vi "Event-MouseWheel.vi"(8 "error in (no error)":errorcluster, 9 "MouseWheelEvent":T1, 10 "EventType":T5=enum."SDL_EVENT_WINDOW_DESTROYED", 11 "DVR Cluster In":T6={"CMD Queue"=refnum, "Config"={"Quit On Last Window Closed"=FALSE, "VSync"=enum."Disabled", "FPS Target"=30.0}, "Ctxt"={"VSync Enabled"=FALSE}, "Metrics"={"Uptime [ms]"=0, "Loop Time [ms]"=0, "Timer [ns]"=0, "Poll Events [ns]"=0, "Dequeue CMD [ns]"=0, "Update Layout [ns]"=0, "Render [ns]"=0}, "Debug"={"Unhandled Events"={}}, "ID To Window"={}, "Window To Handle"={}, "Event Interface"=refnum}) -> (0 "error out":errorcluster, 3 "DVR Cluster Out":T6={"CMD Queue"=refnum, "Config"={"Quit On Last Window Closed"=FALSE, "VSync"=enum."Disabled", "FPS Target"=30.0}, "Ctxt"={"VSync Enabled"=FALSE}, "Metrics"={"Uptime [ms]"=0, "Loop Time [ms]"=0, "Timer [ns]"=0, "Poll Events [ns]"=0, "Dequeue CMD [ns]"=0, "Update Layout [ns]"=0, "Render [ns]"=0}, "Debug"={"Unhandled Events"={}}, "ID To Window"={}, "Window To Handle"={}, "Event Interface"=refnum})   [LabVIEW 2020, in "GLF.lvlib" / "Engine.lvclass"]
uses:
  Engine.lvclass
  EngineEventInterface/EngineEventInterface.lvclass
  Window/Window.lvclass
  Engine.lvclass/Engine.ctl
  <vilib>/Utility/miscctls.llb/LVMapReplaceAction.ctl
  <vilib>/Saukko/LV SDL3/Sources/SDL3/Events/EventType--enum.ctl
  <vilib>/Saukko/LV SDL3/Sources/SDL3/Events/Events.lvlib
  <vilib>/Saukko/LV SDL3/Sources/SDL3/Rect/FPoint--cluster.ctl
  <vilib>/Saukko/LV SDL3/Sources/SDL3/Rect/Rect.lvlib
  VSync--enum.ctl
  Config--cluster.ctl
  Context--cluster.ctl
  Metrics--cluster.ctl
  Command--enum.ctl
  Command--cluster.ctl
  Command--queue.ctl
  <vilib>/Saukko/LV SDL3/Sources/SDL3/Video/WindowID--integer.ctl
  <vilib>/Saukko/LV SDL3/Sources/SDL3/Video/Video.lvlib
  DVR--cluster.ctl
  Debug--cluster.ctl
  <vilib>/Saukko/LV SDL3/Sources/SDL3/Mouse/MouseID--integer.ctl
  <vilib>/Saukko/LV SDL3/Sources/SDL3/Mouse/Mouse.lvlib
  <vilib>/Saukko/LV SDL3/Sources/SDL3/Mouse/MouseWheelDirection--enum.ctl
  <vilib>/Saukko/LV SDL3/Sources/SDL3/Events/MouseWheelEventData--cluster.ctl
  <vilib>/Saukko/LV SDL3/Sources/SDL3/Video/SDL_Window--pointer.ctl
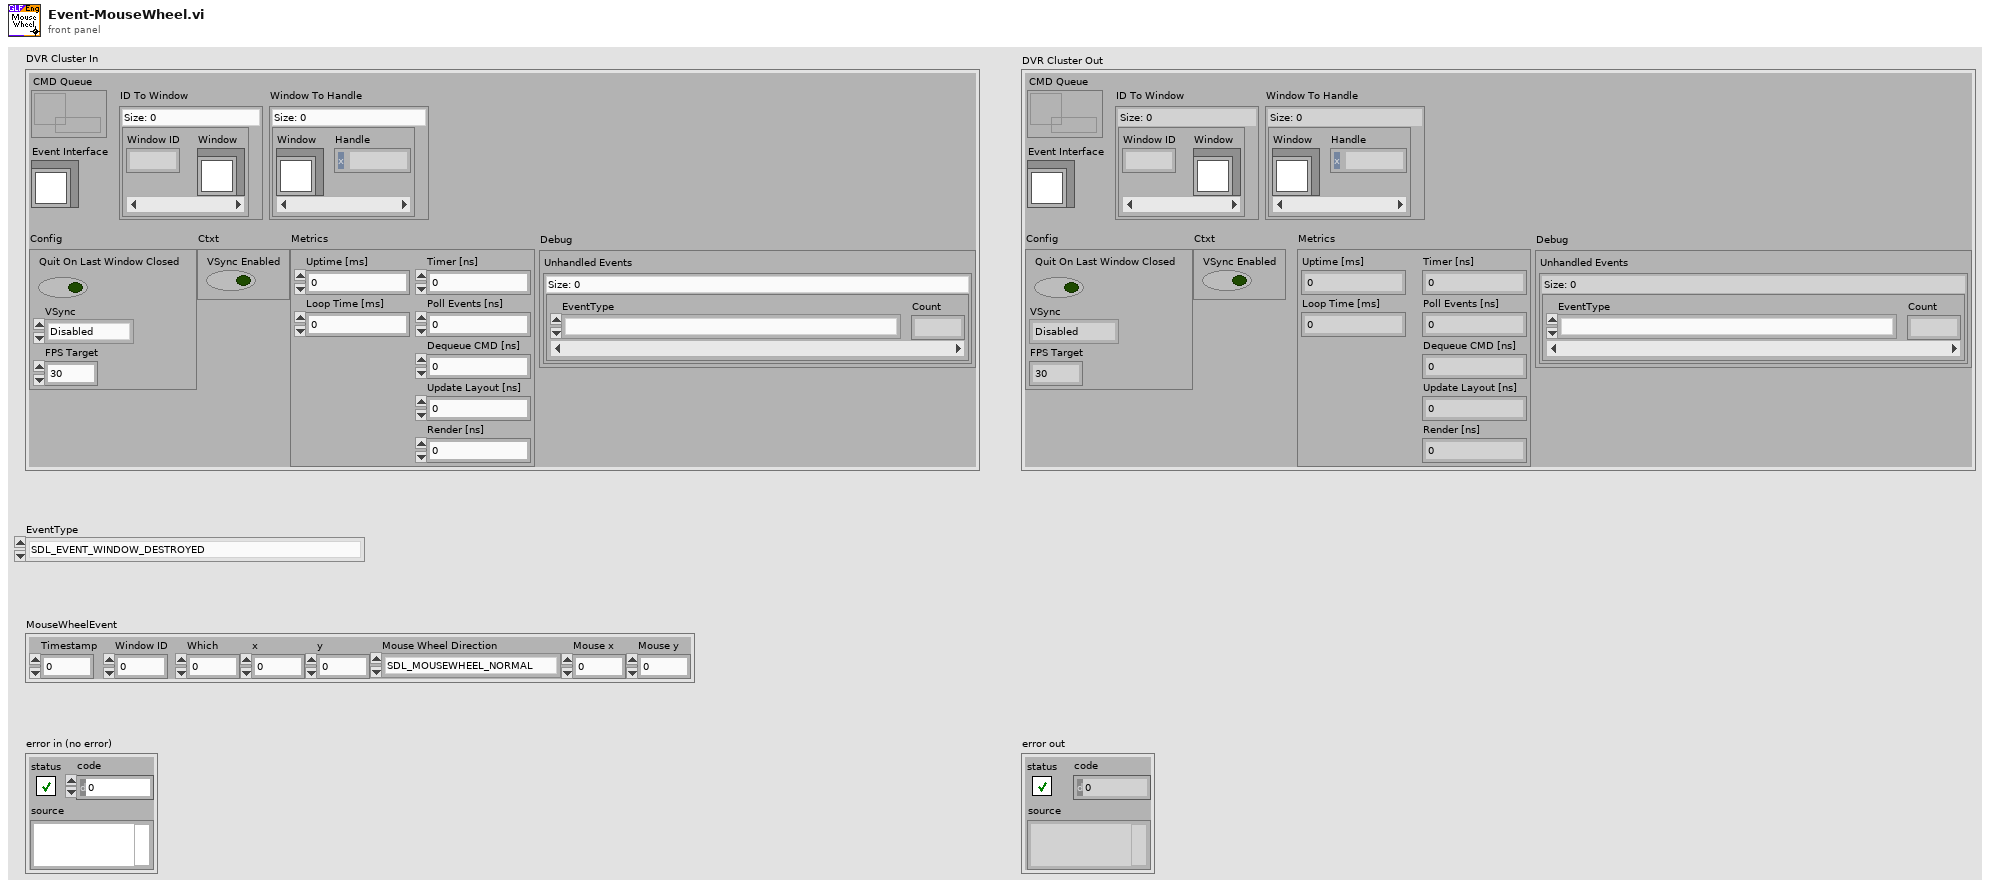
[diagram p1: front panel]
types:
  T1 = typedef "SDL3.lvlib/Events.lvlib/MouseWheelEventData--cluster.ctl" = cluster{"Timestamp":u64, "Window ID":T2, "Which":T3, "x":sgl, "y":sgl, "Mouse Wheel Direction":T4, "Mouse x":sgl, "Mouse y":sgl}
  T2 = typedef "SDL3.lvlib/Video.lvlib/WindowID--integer.ctl" = u32
  T3 = typedef "SDL3.lvlib/Mouse.lvlib/MouseID--integer.ctl" = u32
  T4 = typedef "SDL3.lvlib/Mouse.lvlib/MouseWheelDirection--enum.ctl" = enum32{"SDL_MOUSEWHEEL_NORMAL", "SDL_MOUSEWHEEL_FLIPPED"}
  T5 = typedef "SDL3.lvlib/Events.lvlib/EventType--enum.ctl" = enum16{"LV_NONE", "LV_UNSUPPORTED", "SDL_EVENT_QUIT", "SDL_EVENT_LOCALE_CHANGED", "SDL_EVENT_SYSTEM_THEME_CHANGED", "SDL_EVENT_DISPLAY_ORIENTATION", "SDL_EVENT_DISPLAY_ADDED", "SDL_EVENT_DISPLAY_REMOVED", "SDL_EVENT_DISPLAY_MOVED", "SDL_EVENT_DISPLAY_DESKTOP_MODE_CHANGED", "SDL_EVENT_DISPLAY_CURRENT_MODE_CHANGED", "SDL_EVENT_DISPLAY_CONTENT_SCALE_CHANGED", "SDL_EVENT_WINDOW_SHOWN", "SDL_EVENT_WINDOW_HIDDEN", "SDL_EVENT_WINDOW_EXPOSED", "SDL_EVENT_WINDOW_MOVED", "SDL_EVENT_WINDOW_RESIZED", "SDL_EVENT_WINDOW_PIXEL_SIZE_CHANGED", "SDL_EVENT_WINDOW_METAL_VIEW_RESIZED", "SDL_EVENT_WINDOW_MINIMIZED", "SDL_EVENT_WINDOW_MAXIMIZED", "SDL_EVENT_WINDOW_RESTORED", "SDL_EVENT_WINDOW_MOUSE_ENTER", "SDL_EVENT_WINDOW_MOUSE_LEAVE", "SDL_EVENT_WINDOW_FOCUS_GAINED", "SDL_EVENT_WINDOW_FOCUS_LOST", "SDL_EVENT_WINDOW_CLOSE_REQUESTED", "SDL_EVENT_WINDOW_HIT_TEST", "SDL_EVENT_WINDOW_ICCPROF_CHANGED", "SDL_EVENT_WINDOW_DISPLAY_CHANGED", "SDL_EVENT_WINDOW_DISPLAY_SCALE_CHANGED", "SDL_EVENT_WINDOW_SAFE_AREA_CHANGED", "SDL_EVENT_WINDOW_OCCLUDED", "SDL_EVENT_WINDOW_ENTER_FULLSCREEN", "SDL_EVENT_WINDOW_LEAVE_FULLSCREEN", "SDL_EVENT_WINDOW_DESTROYED", "SDL_EVENT_WINDOW_HDR_STATE_CHANGED", "SDL_EVENT_KEY_DOWN", "SDL_EVENT_KEY_UP", "SDL_EVENT_TEXT_EDITING", "SDL_EVENT_TEXT_INPUT", "SDL_EVENT_KEYMAP_CHANGED", "SDL_EVENT_KEYBOARD_ADDED", "SDL_EVENT_KEYBOARD_REMOVED", "SDL_EVENT_TEXT_EDITING_CANDIDATES", "SDL_EVENT_MOUSE_MOTION", "SDL_EVENT_MOUSE_BUTTON_DOWN", "SDL_EVENT_MOUSE_BUTTON_UP", "SDL_EVENT_MOUSE_WHEEL", "SDL_EVENT_MOUSE_ADDED", "SDL_EVENT_MOUSE_REMOVED", "SDL_EVENT_JOYSTICK_AXIS_MOTION", "SDL_EVENT_JOYSTICK_BALL_MOTION", "SDL_EVENT_JOYSTICK_HAT_MOTION", "SDL_EVENT_JOYSTICK_BUTTON_DOWN", "SDL_EVENT_JOYSTICK_BUTTON_UP", "SDL_EVENT_JOYSTICK_ADDED", "SDL_EVENT_JOYSTICK_REMOVED", "SDL_EVENT_JOYSTICK_BATTERY_UPDATED", "SDL_EVENT_JOYSTICK_UPDATE_COMPLETE", "SDL_EVENT_GAMEPAD_AXIS_MOTION", "SDL_EVENT_GAMEPAD_BUTTON_DOWN", "SDL_EVENT_GAMEPAD_BUTTON_UP", "SDL_EVENT_GAMEPAD_ADDED", "SDL_EVENT_GAMEPAD_REMOVED", "SDL_EVENT_GAMEPAD_REMAPPED", "SDL_EVENT_GAMEPAD_TOUCHPAD_DOWN", "SDL_EVENT_GAMEPAD_TOUCHPAD_MOTION", "SDL_EVENT_GAMEPAD_TOUCHPAD_UP", "SDL_EVENT_GAMEPAD_SENSOR_UPDATE", "SDL_EVENT_GAMEPAD_UPDATE_COMPLETE", "SDL_EVENT_GAMEPAD_STEAM_HANDLE_UPDATED", "SDL_EVENT_FINGER_DOWN", "SDL_EVENT_FINGER_UP", "SDL_EVENT_FINGER_MOTION", "SDL_EVENT_CLIPBOARD_UPDATE", "SDL_EVENT_DROP_FILE", "SDL_EVENT_DROP_TEXT", "SDL_EVENT_DROP_BEGIN", "SDL_EVENT_DROP_COMPLETE", "SDL_EVENT_DROP_POSITION", "SDL_EVENT_AUDIO_DEVICE_ADDED", "SDL_EVENT_AUDIO_DEVICE_REMOVED", "SDL_EVENT_AUDIO_DEVICE_FORMAT_CHANGED", "SDL_EVENT_SENSOR_UPDATE", "SDL_EVENT_PEN_PROXIMITY_IN", "SDL_EVENT_PEN_PROXIMITY_OUT", "SDL_EVENT_PEN_DOWN", "SDL_EVENT_PEN_UP", "SDL_EVENT_PEN_BUTTON_DOWN", "SDL_EVENT_PEN_BUTTON_UP", "SDL_EVENT_PEN_MOTION", "SDL_EVENT_PEN_AXIS", "SDL_EVENT_CAMERA_DEVICE_ADDED", "SDL_EVENT_CAMERA_DEVICE_REMOVED", "SDL_EVENT_CAMERA_DEVICE_APPROVED", "SDL_EVENT_CAMERA_DEVICE_DENIED", "SDL_EVENT_RENDER_TARGETS_RESET", "SDL_EVENT_RENDER_DEVICE_RESET", "SDL_EVENT_POLL_SENTINEL", "SDL_EVENT_USER"}
  T6 = typedef "GLF.lvlib/Engine.lvclass/DVR--cluster.ctl" = cluster{"CMD Queue":T7, "Config":T8, "Ctxt":T10, "Metrics":T11, "Debug":T12, "ID To Window":map{T2, refnum<class "Window.lvclass">}, "Window To Handle":map{refnum<class "Window.lvclass">, T13}, "Event Interface":refnum<class "EngineEventInterface.lvclass">}
  T7 = typedef "GLF.lvlib/Engine.lvclass/Command--queue.ctl" = refnum<queue>
  T8 = typedef "GLF.lvlib/Engine.lvclass/Config--cluster.ctl" = cluster{"Quit On Last Window Closed":bool, "VSync":T9, "FPS Target":dbl}
  T9 = typedef "GLF.lvlib/Engine.lvclass/VSync--enum.ctl" = enum16{"Disabled", "Enabled", "Adaptative"}
  T10 = typedef "GLF.lvlib/Engine.lvclass/Context--cluster.ctl" = cluster{"VSync Enabled":bool}
  T11 = typedef "GLF.lvlib/Engine.lvclass/Metrics--cluster.ctl" = cluster{"Uptime [ms]":u64, "Loop Time [ms]":u64, "Timer [ns]":u64, "Poll Events [ns]":u64, "Dequeue CMD [ns]":u64, "Update Layout [ns]":u64, "Render [ns]":u64}
  T12 = typedef "GLF.lvlib/Engine.lvclass/Debug--cluster.ctl" = cluster{"Unhandled Events":map{T5, u64}}
  T13 = typedef "SDL3.lvlib/Video.lvlib/SDL_Window--pointer.ctl" = i64
  T14 = typedef "LVMapReplaceAction.ctl" = enum32{"Modify Entry only if found", "Add or Modify Entry", "Delete Entry"}
  T15 = typedef "SDL3.lvlib/Rect.lvlib/FPoint--cluster.ctl" = cluster{"x":sgl, "y":sgl}
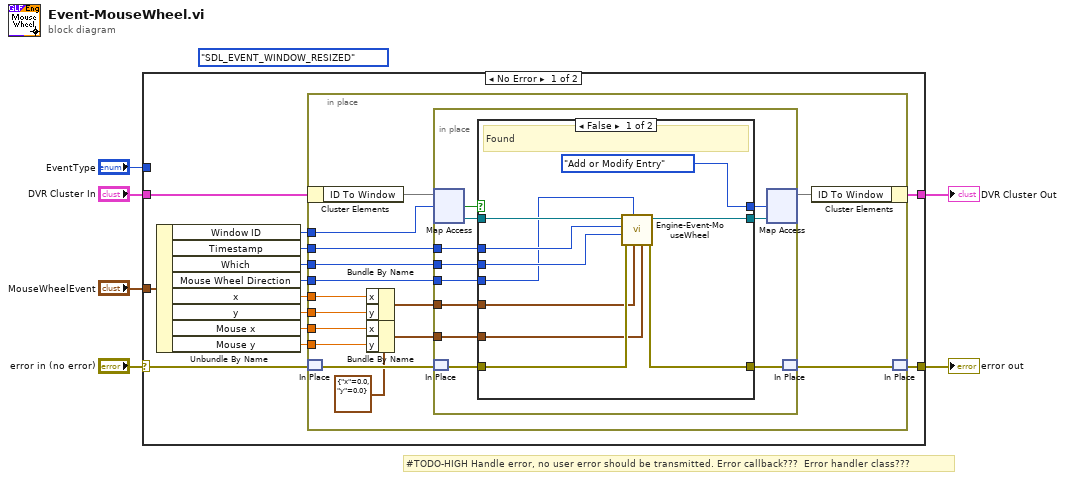
[diagram p0: block diagram]
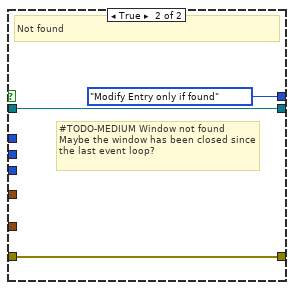
[diagram p2: hidden frame]
diagram:
  (unwired) EventType--enum."SDL_EVENT_WINDOW_RESIZED" ("EventType")
  # "#TODO-HIGH Handle error, no user error should be transmitted. Error callback???  Error handler class???"
  n1 = case shown="No Error" "error in (no error)" {
    selector: "error in (no error)" -> [w16 w60]
    tunnel: [w13 w60] -> w5
    tunnel: [w14 w59] -> w3
    tunnel: "DVR Cluster In" -> [w18 w59]
    tunnel: "MouseWheelEvent" -> [w19 _]
    tunnel: "EventType" -> [_ _]
    frame No Error {
      n2 = Unbundle By Name(w19) -> ("Window ID"=w17:T2, "Timestamp"=w15:u64, "Which"=w12:T3, "Mouse Wheel Direction"=w11:T4, "x"=w7:sgl, "y"=w10:sgl, "Mouse x"=w9:sgl, "Mouse y"=w8:sgl)
      n3 = in-place {
        in-place-border: w17 -> [w33]
        in-place-border: w15 -> [w30]
        in-place-border: w12 -> [w28]
        in-place-border: w11 -> [w27]
        in-place-border: w10 -> [w25]
        in-place-border: w9 -> [w24]
        in-place-border: w8 -> [w23]
        in-place-border: w7 -> [w26]
        w22 = T15 {"x"=0.0, "y"=0.0} ("FPoint")
        n4 = in-place-cluster #1(w18) -> ("ID To Window"=w34:map{T2, refnum<class "Window.lvclass">})
        n5 = in-place-match #2(w16) -> (w32:errorcluster)
        n6 = Bundle By Name(cluster=w22, "x"=w26, "y"=w25) -> (w21:T15)
        n7 = Bundle By Name(cluster=w22, "x"=w24, "y"=w23) -> (w20:T15)
        n8 = in-place {
          in-place-border: w30 -> [w39]
          in-place-border: w28 -> [w38]
          in-place-border: w27 -> [w37]
          in-place-border: w21 -> [w36]
          in-place-border: w20 -> [w35]
          n9 = in-place-map #3(w34, w33) -> (w44:refnum<class "Window.lvclass">, w45:bool)  [unwired: 1 in]
          n10 = in-place-match #4(w32) -> (w42:errorcluster)
          n11 = case shown="False" w45 {
            tunnel: w44 -> [w55 w56]
            tunnel: [LVMapReplaceAction."Add or Modify Entry" ("Replace Action") LVMapReplaceAction."Modify Entry only if found" ("Replace Action")] -> w43
            tunnel: [w46 w57] -> w41
            tunnel: w42 -> [w54 w57]
            tunnel: [w51 w56] -> w40
            tunnel: w39 -> [w53 _]
            tunnel: w38 -> [w52 _]
            tunnel: w37 -> [w48 _]
            tunnel: w36 -> [w50 _]
            tunnel: w35 -> [w49 _]
            frame False {
              # "Found"
              n12 = call "Engine-Event-MouseWheel.vi"("Mouse Position"=w49, "Wheel"=w50, "Mouse Wheel Direction"=w48, "error in (no error)"=w54, "Which"=w52, "Timestamp"=w53, "GLF Window in"=w55) -> ("error out"=w46:errorcluster, "GLF Window out"=w51:refnum<class "Window.lvclass">)  [unwired: 3 in]
            }
            frame True {
              # "#TODO-MEDIUM Window not found\nMaybe the window has been closed since the last event loop?"
              # "Not found"
            }
          }
          n13 = in-place-map #3(w40, w43) -> (w29:map{T2, refnum<class "Window.lvclass">})  [unwired: 2 out]
          n14 = in-place-match #4(w41) -> (w31:errorcluster)
        }
        n15 = in-place-cluster #1("ID To Window"=w29) -> (w14:T6)
        n16 = in-place-match #2(w31) -> (w13:errorcluster)
      }
    }
    frame Error {
    }
  }
  "error out" <- w5
  "DVR Cluster Out" <- w3
